vi "axex_open_file.vi"(7 "open active workbook (False)":bool, 8 "error in":errorcluster, 9 "window state (unchanged)":T2=enum."Don't change", 10 "reload from file (False)":bool, 11 "excel file path (full)":path) -> (0 "error out":errorcluster, 3 "AX Excel instance out":T1)   [LabVIEW 2020, in "AX Excel.lvlib"]
doc: "Call this to open given Excel file. Use 'reload' option to reload Excel file from disk discarding all possible changes if the file was already opened in Excel. Use 'window state' input to change state of Excel application window."
uses:
  AX Excel.lvlib
  axex_window_state.ctl
  axex_instance.ctl
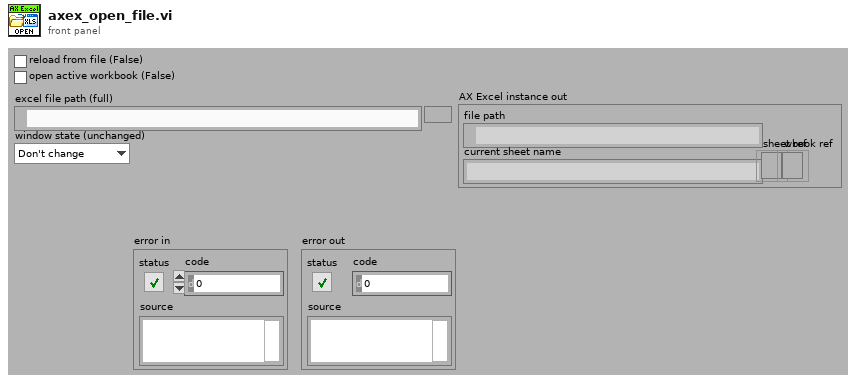
[diagram p1: front panel]
types:
  T1 = typedef "AX Excel.lvlib/axex_instance.ctl" = cluster{"file path":path, "current sheet name":string, "sheet ref":refnum<k7>, "wbook ref":refnum<k7>}
  T2 = typedef "AX Excel.lvlib/axex_window_state.ctl" = enum16{"Minimized", "Maximized", "Normal", "Don't change"}
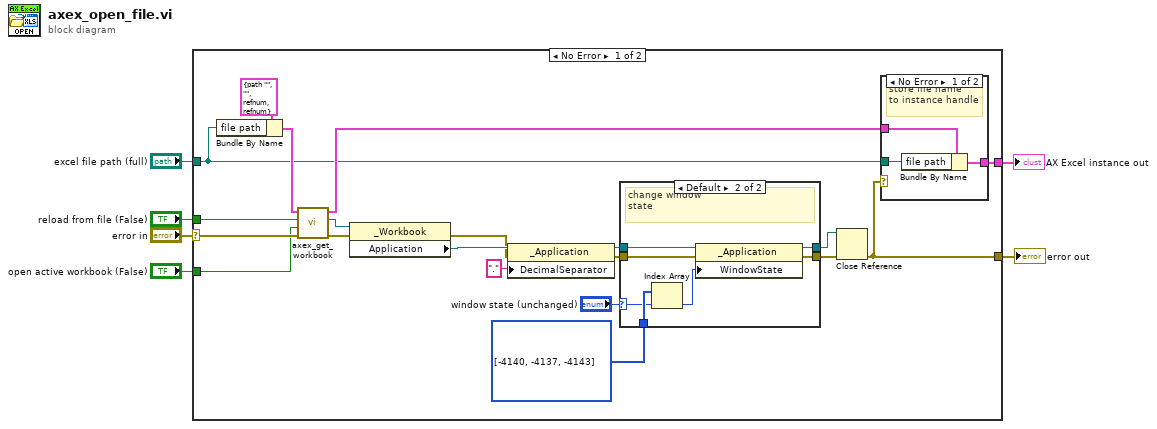
[diagram p0: block diagram]
diagram:
  n1 = case shown="No Error" "error in" {
    selector: "error in" -> [w8 w40]
    tunnel: "reload from file (False)" -> [w25 _]
    tunnel: [w17 _] -> w5
    tunnel: [w16 w40] -> w4
    tunnel: "excel file path (full)" -> [w11 _]
    tunnel: "open active workbook (False)" -> [w7 _]
    frame No Error {
      n2 = Bundle By Name(cluster=T1 {"file path"=path "", "current sheet name"="", "sheet ref"=refnum, "wbook ref"=refnum} ("SX Excel instance"), "file path"=w11) -> (w14:T1)
      n3 = call "axex_get_workbook.vi"("error in"=w8, "open active workbook (False)"=w7, "reload from file (False)"=w25, "AX Excel instance in"=w14) -> ("error out"=w26:errorcluster, "excel workbook"=w13:refnum<k7>, "AX Excel instance out"=w12:T1)  [unwired: 5 in]
      n4 = property class="_Workbook"(reference=w13, error in=w26) -> (error out=w9:errorcluster, "Application"=w24:refnum<k7>)  [unwired: 1 out]
      n5 = property class="_Application"(reference=w24, error in=w9, "DecimalSeparator"=".") -> (reference out=w21:refnum<k7>, error out=w22:errorcluster)
      n6 = case shown="Default" "window state (unchanged)" {
        selector: "window state (unchanged)" -> [_ w33]
        tunnel: w22 -> [w32 w39]
        tunnel: w21 -> [w31 w38]
        tunnel: [w32 w37] -> w19
        tunnel: [w31 w36] -> w18
        tunnel: i32[] [-4140, -4137, -4143] -> [_ w34]
        frame "Don't change" {
        }
        frame Default {
          # "change window\nstate"
          n7 = Index Array(array=w34, index=w33) -> (element=w35:i32)
          n8 = property class="_Application"(reference=w38, error in=w39, "WindowState"=w35) -> (reference out=w36:refnum<k7>, error out=w37:errorcluster)
        }
      }
      n9 = Close Reference(reference=w18, error in (no error)=w19) -> (error out=w16:errorcluster)
      n10 = case shown="No Error" w16 {
        tunnel: [w29 w30] -> w17
        tunnel: w11 -> [w28 _]
        tunnel: w12 -> [w27 w30]
        frame No Error {
          # "store file name\nto instance handle"
          n11 = Bundle By Name(cluster=w27, "file path"=w28) -> (w29:T1)
        }
        frame Error {
        }
      }
    }
    frame Error {
    }
  }
  "error out" <- w4
  "AX Excel instance out" <- w5
